vi "Boolean Update.vi"(8 "error in (no error)":errorcluster, 9 "Control in":refnum<vi>, 11 "Material-Scheme.lvclass":refnum<class "Material-Scheme.lvclass">) -> (0 "error out":errorcluster)   [LabVIEW 2021, in "TSC Material Theme.lvlib" / "Material-Scheme.lvclass"]
doc: "Set the boolean scheme - will be the most involved of the control types\n\n<b>Code Developed By:</b>\nTechnology Service Corporation\nwww.tsc.com/atcs\n\nDeveloper:\nDaniel Coons"
uses:
  Material-Scheme.lvclass
  Material-Scheme.lvclass/Material-Scheme.ctl
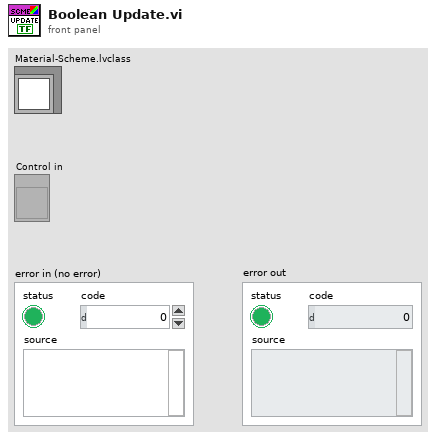
[diagram p1: front panel]
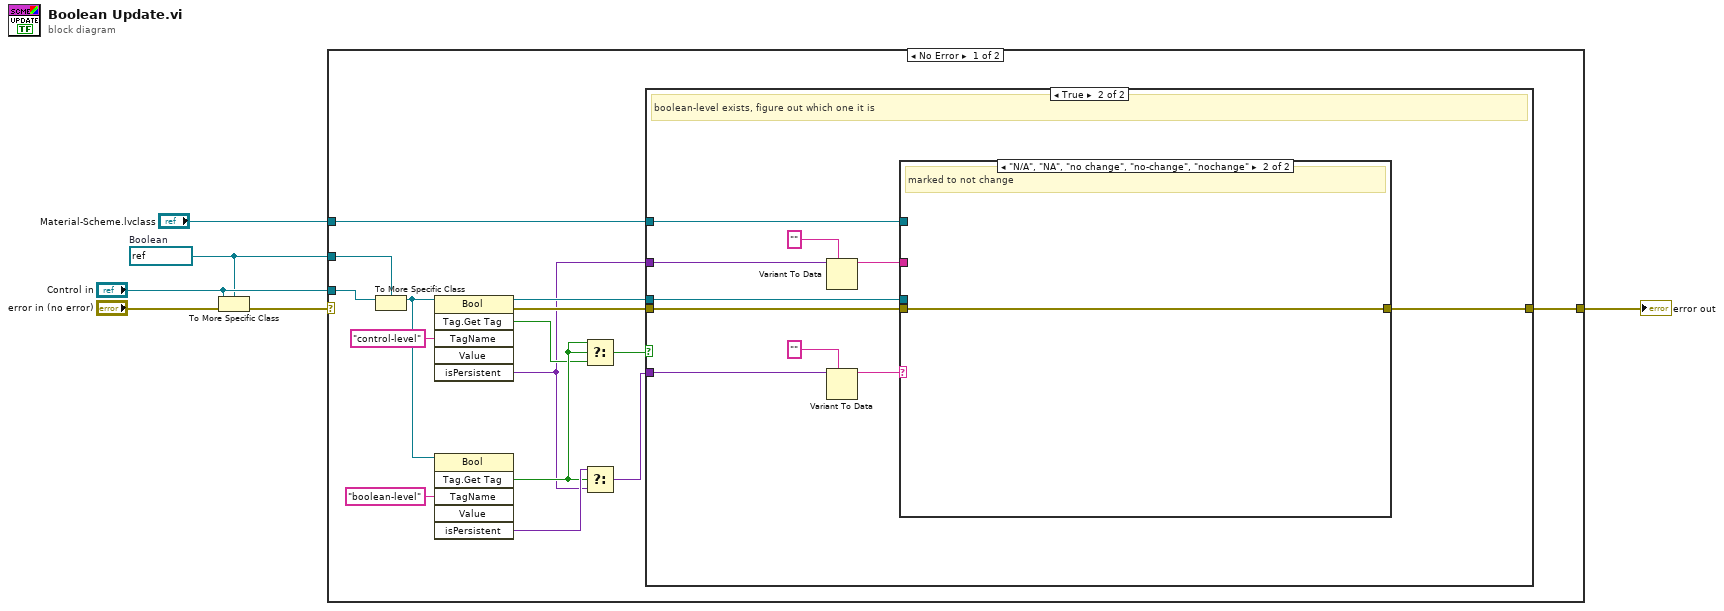
[diagram p0: block diagram]
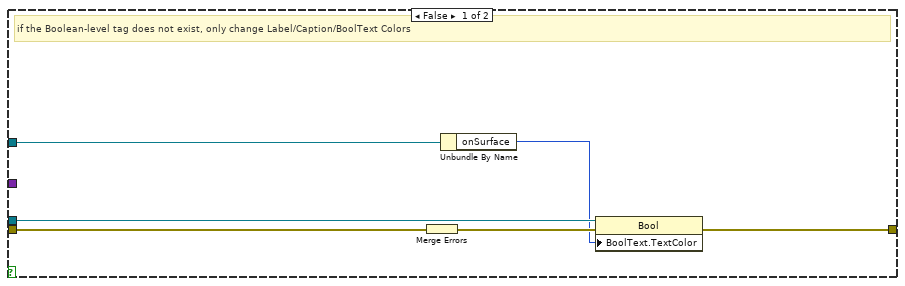
[diagram p2: hidden frame]
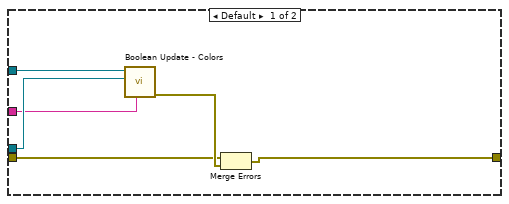
[diagram p3: hidden frame]
diagram:
  w3 = refnum<vi> refnum  # Boolean
  n1 = To More Specific Class(target class=w3, reference="Control in", error in="error in (no error)") -> (error out=w5:errorcluster)  [unwired: 1 out]
  n2 = case shown="No Error" w5 {
    selector: w5 -> [_ w45]
    tunnel: "Control in" -> [w21 _]
    tunnel: w3 -> [w20 _]
    tunnel: [w16 w45] -> w2
    tunnel: "Material-Scheme.lvclass" -> [w17 _]
    frame No Error {
      n3 = To More Specific Class(target class=w20, reference=w21) -> (specific class reference=w13:refnum<vi>)  [unwired: 1 in, 1 out]
      n4 = invoke class="Bool" method="Tag.Get Tag"(reference=w13, "TagName"="control-level" ("Tag Name")) -> (reference out=w15:refnum<vi>, error out=w18:errorcluster, "GetTag"=w9:bool, "isPersistent"=w7:variant)  [unwired: 4 in, 2 out]
      n5 = invoke class="Bool" method="Tag.Get Tag"(reference=w13, "TagName"="boolean-level" ("Tag Name")) -> ("GetTag"=w10:bool, "isPersistent"=w12:variant)  [unwired: 4 in, 4 out]
      n6 = Select(t=w10, s=w10, f=w9) -> (s? t:f=w8:bool)
      n7 = Select(t=w12, s=w10, f=w7) -> (s? t:f=w11:variant)
      n8 = case shown="True" w8 {
        tunnel: w18 -> [w27 w33]
        tunnel: w11 -> [_ w28]
        tunnel: w15 -> [w24 w34]
        tunnel: w17 -> [w23 w35]
        tunnel: [w26 w32] -> w16
        tunnel: w7 -> [_ w30]
        frame False {
          # "if the Boolean-level tag does not exist, only change Label/Caption/BoolText Colors"
          n9 = Merge Errors(w27) -> (w25:errorcluster)
          n10 = Unbundle By Name(w23) -> ("onSurface"=w22:u32)
          n11 = property class="Bool"(reference=w24, error in=w25, "BoolText.TextColor"=w22) -> (error out=w26:errorcluster)  [unwired: 1 out]
        }
        frame True {
          # "boolean-level exists, figure out which one it is"
          n12 = Variant To Data(type="", Variant=w30) -> (data=w29:string)  [unwired: 1 in, 1 out]
          n13 = Variant To Data(type="", Variant=w28) -> (data=w36:string)  [unwired: 1 in, 1 out]
          n14 = case shown="\"N/A\", \"NA\", \"no change\", \"no-change\", \"nochange\"" w36 {
            tunnel: w35 -> [w39 _]
            tunnel: w34 -> [w40 _]
            tunnel: w33 -> [w41 w44]
            tunnel: [w43 w44] -> w32
            tunnel: w29 -> [w38 _]
            frame Default {
              n15 = call "Boolean Update - Colors.vi"("control-level"=w38, "Bool Refnum"=w40, "Material-Scheme in"=w39) -> ("error out"=w42:errorcluster)  [unwired: 5 in, 3 out]
              n16 = Merge Errors(w41, w42) -> (w43:errorcluster)
            }
            frame "N/A", "NA", "no change", "no-change", "nochange" {
              # "marked to not change"
            }
          }
        }
      }
    }
    frame Error {
    }
  }
  "error out" <- w2
